vi "LPC set power.vi"(8 "error in (no error)":errorcluster, 10 "power":dbl[unit]=0.005, 11 "VISA resource name":refnum<visa-resource-name>="GPIB0::8::INSTR") -> (0 "error out":errorcluster, 3 "VISA resource name out":refnum<visa-resource-name>)   [LabVIEW 2015, in "BEOC LPC.lvlib"]
doc: "Sets the power of the LPC (laser power controller)."
uses:
  BEOC LPC.lvlib
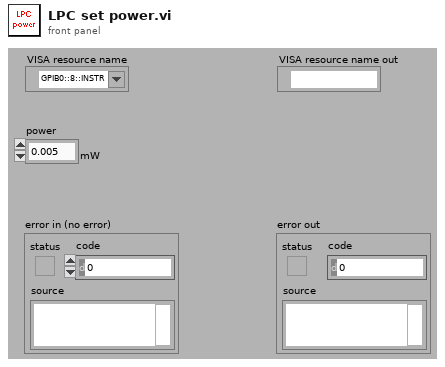
[diagram p1: front panel]
types:
  T1 = typedef "Semaphore RefNum" = refnum<k1>
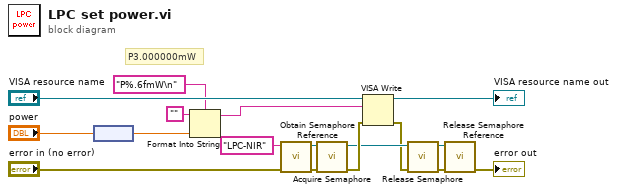
[diagram p0: block diagram]
diagram:
  # "P3.000000mW"
  n1 = node("power") -> (w1:dbl)
  n2 = Format Into String(format string="P%.6fmW\n", initial string="", w1) -> (resulting string=w13:string)  [unwired: 1 in, 1 out]
  n3 = call <vilib>:"Obtain Semaphore Reference.vi"("error in (no error)"="error in (no error)", "name (unnamed)"="LPC-NIR") -> ("error out"=w9:errorcluster, "semaphore"=w8:T1)  [unwired: 1 in, 3 out]
  n4 = call <vilib>:"Acquire Semaphore.vi"("error in (no error)"=w9, "semaphore"=w8) -> ("error out"=w5:errorcluster, "semaphore out"=w4:T1)  [unwired: 1 in, 3 out]
  n5 = VISA Write(VISA resource name="VISA resource name", write buffer=w13, error in (no error)=w5) -> (VISA resource name out=→"VISA resource name out":refnum<visa-resource-name>, error out=w3:errorcluster)  [unwired: 1 out]
  n6 = call <vilib>:"Release Semaphore.vi"("error in (no error)"=w3, "semaphore"=w4) -> ("error out"=w7:errorcluster, "semaphore out"=w6:T1)  [unwired: 4 out]
  n7 = call <vilib>:"Release Semaphore Reference.vi"("error in (no error)"=w7, "semaphore"=w6) -> ("error out"=→"error out":errorcluster)  [unwired: 9 out]
